vi "Read Example.vi"(0 "Source Address":u8=228 format="%.0x", 1 "Read Timeout (ms)":u32=500, 2 "Device Selected":i32, 5 "Expected Command":string=".*", 7 "Expected Data":string=".*", 9 "Expected Source":string=".*", 11 "Error In":errorcluster, 13 "# of Tries":u8=5 min=1) -> (4 "Data Returned":string, 6 "Coverted Data Out":T1 {"CRC" format="%04x"; "Length" format="%02x"; "Command" format="%02x"; "Destination" format="%02x"; "Source" format="%02x"}, 15 "Error Out":errorcluster)   [LabVIEW 2016]
doc: "This standalone VI reads the next message on the GEA2 bus OR waits until it receives a message with the command or data you specify. (.* = anything)"
uses:
  LabVIEW_GEA2_Toolkit.lvlibp/type defs/Data Out.ctl
  LabVIEW_GEA2_Toolkit.lvlibp
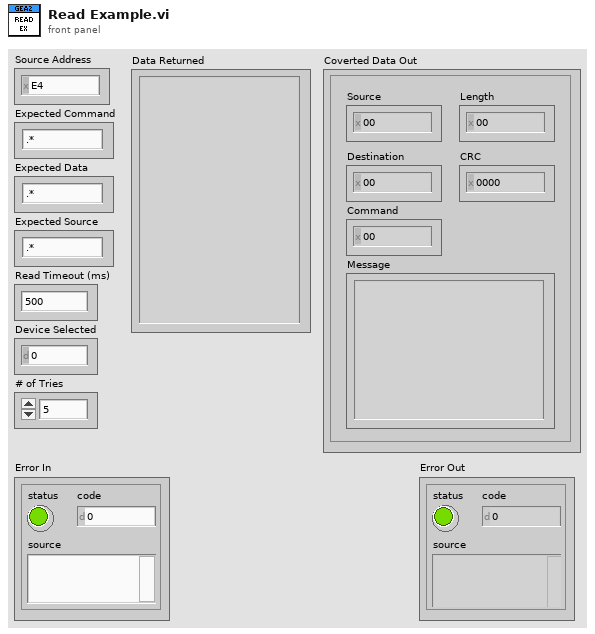
[diagram p1: front panel]
types:
  T1 = typedef "LabVIEW_GEA2_Toolkit.lvlibp/Data Out.ctl" = cluster{"Source":u8, "Destination":u8, "Command":u8, "Length":u8, "CRC":u16, "Message":string}
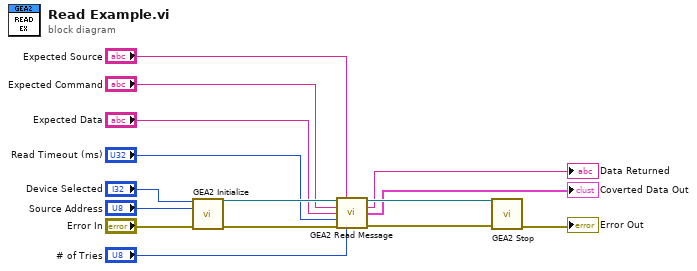
[diagram p0: block diagram]
diagram:
  n1 = call "GEA2 Initialize.vi"("Board Index"="Device Selected", "Source Address"="Source Address", "error in"="Error In") -> ("GEA2 Reference Out"=w13:refnum<k24>, "error out"=w12:errorcluster)  [unwired: 10 in, 1 out]
  n2 = call "GEA2 Read Message.vi"("GEA2 Reference In"=w13, "Expected Source"="Expected Source", "Expected Command"="Expected Command", "Expected Data"="Expected Data", "Timeout (ms)"="Read Timeout (ms)", "Error In"=w12, "# of Tries"="# of Tries") -> ("GEA2 Reference Out"=w14:refnum<k24>, "Raw Data Out"=→"Data Returned":string, "Coverted Data Out"=→"Coverted Data Out":T1, "Error Out"=w15:errorcluster)  [unwired: 5 in]
  n3 = call "GEA2 Stop.vi"("GEA2 Reference In"=w14, "Error In"=w15) -> ("Error Out"=→"Error Out":errorcluster)  [unwired: 13 in]
